vi "Convert I2C Messages.vi"(8 "error in (no error)":errorcluster, 11 "Fetched I2C Messages Ref":refnum<vi>) -> (0 "error out":errorcluster, 3 "I2C Messages":string[][](array[string]))   [LabVIEW 2025, in "I2C Bus Monitor UI.lvlib"]
uses:
  I2C Bus Monitor UI.lvlib
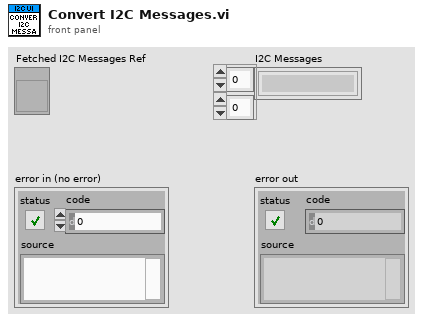
[diagram p1: front panel]
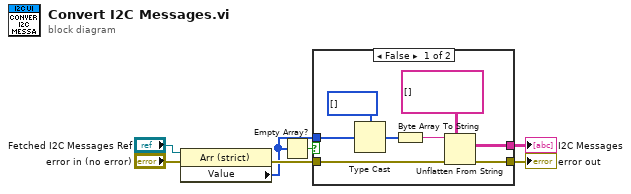
[diagram p0: block diagram]
diagram:
  n1 = property class="Arr (strict)"(reference="Fetched I2C Messages Ref", error in="error in (no error)") -> (error out=w4:errorcluster, "Value"=w2:u64[])  [unwired: 1 out]
  n2 = Empty Array?(array=w2) -> (empty?=w1:bool)
  n3 = case shown="False" w1 {
    tunnel: [w11 w16] -> w6
    tunnel: [w10 _] -> w5
    tunnel: w4 -> [w9 w16]
    tunnel: w2 -> [w8 _]
    frame False {
      n4 = Type Cast(type=u8[] [] ("unsigned byte array"), x=w8) -> (*(type *) &x=w14:u8[])
      n5 = Byte Array To String(unsigned byte array=w14) -> (string=w12:string)
      n6 = Unflatten From String(type=string[][] [] ("Fetched I2C Messages"), binary string=w12, error in (no error)=w9) -> (value=w10:string[][], error out=w11:errorcluster)  [unwired: 2 in, 1 out]
    }
    frame True {
    }
  }
  "error out" <- w6
  "I2C Messages" <- w5
